vi "LVClass_Camera Get parameters whose differ from CameraSet.vi"(0 "Camera in":refnum<class "Camera.lvclass">, 5 "CameraSet in":refnum<class "CameraSet.lvclass">, 11 "error in (no error)":errorcluster) -> (4 "Camera out":refnum<class "Camera.lvclass">, 6 "CameraSet out":refnum<class "CameraSet.lvclass">, 12 "nb_nonequals_settable_connection_params":i32, 13 "nb_nonequals_onfly_settable_params":i32, 14 "nb_nonequal_settable_params":i32, 15 "error out":errorcluster)   [LabVIEW 2020, in "Camera.lvclass"]
doc: "Load and apply camera parameters from a CameraSet object.\n\n<B>CameraIn</B> : Camera object.\n<B>CameraOut</B> : Camera object.\n<B>CameraSet</B> : CameraSet object.\n<B>nb_nonequal_settable_params</B> : number of settable parameters whose values differ.\n<B>nb_nonequals_onfly_settable_params</B> : number of onfly settable parameters whose values differ.\n<B>nb_nonequals_settable_connection_params</B> : number of settable connection parameters whose values differ."
uses:
  Camera.lvclass
  CameraSet.lvclass
  Camera.lvclass/Camera.ctl
  LVClass_CameraSet Read CameraSet.vi
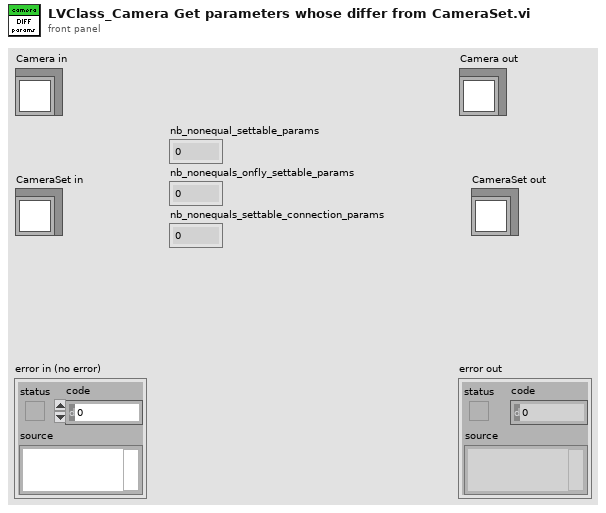
[diagram p1: front panel]
types:
  T1 = typedef "ClassID.ctl" = i64
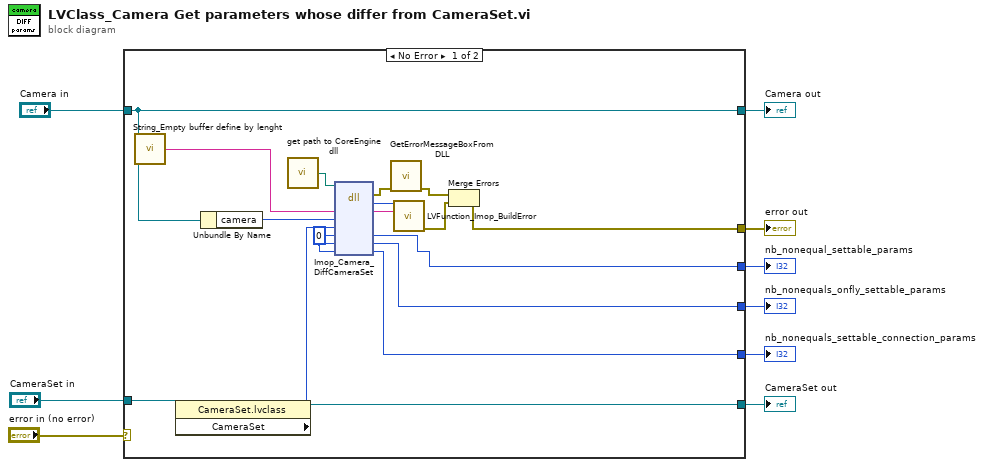
[diagram p0: block diagram]
diagram:
  n1 = case shown="No Error" "error in (no error)" {
    selector: "error in (no error)" -> [_ w28]
    tunnel: [w15 w28] -> w8
    tunnel: [w25 w27] -> w6
    tunnel: "Camera in" -> [w25 w27]
    tunnel: [w16 _] -> w5
    tunnel: "CameraSet in" -> [w17 _]
    tunnel: [w13 _] -> w3
    tunnel: [w12 _] -> w2
    tunnel: [w11 _] -> w1
    frame No Error {
      w10 = 0 ("nb_nonequal_settable_params")
      n2 = call "String_Empty buffer define by lenght.vi"() -> ("Empty buffer"=w26:string)  [unwired: 1 in]
      n3 = property class="CameraSet.lvclass"(reference=w17) -> (reference out=w16:refnum<class "CameraSet.lvclass">, "CameraSet"=w14:T1)  [unwired: 1 in, 1 out]
      n4 = Unbundle By Name(w25) -> ("camera"=w24:T1)
      n5 = call "get path to CoreEngine dll.vi"() -> ("path to c_interface_vc100.dll"=w21:path)  [unwired: 12 in, 3 out]
      n6 = dll-call lib="D:/soft/HASO_v3/SVN_trunk/ImOpCoreEngine4_LV2011/DLLs/c_interface_vc100.dll" fn="Imop_Camera_DiffCameraSet"(path in=w21, "message"=w26, "camera"=w24, "CameraSet"=w14, "nb_nonequal_settable_params"=w10, "nb_nonequals_onfly_settable_params"=w10, "nb_nonequals_settable_connection_params"=w10) -> (error out=w20:errorcluster, "return type"=w22:i32, "message"=w23:string, "nb_nonequal_settable_params"=w13:i32, "nb_nonequals_onfly_settable_params"=w12:i32, "nb_nonequals_settable_connection_params"=w11:i32)  [unwired: 4 in, 1 out]
      n7 = call "GetErrorMessageBoxFromDLL.vi"("error IN"=w20) -> ("error OUT"=w19:errorcluster)  [unwired: 10 in]
      n8 = call "LVFunction_Imop_BuildError.vi"("code"=w22, "String to Prepend to source (\"\")"=w23) -> ("error out"=w18:errorcluster)  [unwired: 13 in]
      n9 = Merge Errors(w19, w18) -> (w15:errorcluster)
    }
    frame Error {
    }
  }
  "error out" <- w8
  "Camera out" <- w6
  "CameraSet out" <- w5
  "nb_nonequal_settable_params" <- w3
  "nb_nonequals_onfly_settable_params" <- w2
  "nb_nonequals_settable_connection_params" <- w1
